vi "GetPathFromPathCtrl.vi"(11 "path ref in":refnum<vi>) -> (2 "result":path, 3 "path ref out":refnum<vi>)   [LabVIEW 2018, in "Library-Ctrl.lvlib"]
uses:
  Library-Ctrl.lvlib
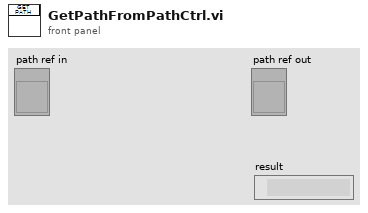
[diagram p1: front panel]
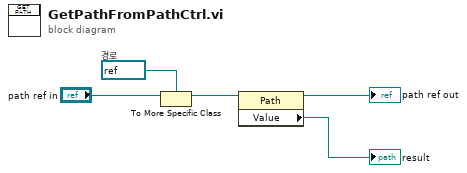
[diagram p0: block diagram]
diagram:
  w4 = refnum<vi> refnum  # 경로
  n1 = To More Specific Class(target class=w4, reference="path ref in") -> (specific class reference=w3:refnum<vi>)  [unwired: 1 in, 1 out]
  n2 = property class="Path"(reference=w3) -> (reference out=→"path ref out":refnum<vi>, "Value"=→"result":path)  [unwired: 1 in, 1 out]
